vi "Assymetric_Arbitrary_Wave.vi"(9 "Time Ratios":dbl[](array[numeric]), 10 "Ub":dbl=1.0, 11 "samples":i32=128) -> (1 "offset":dbl, 2 "amplitude":dbl, 3 "Arbitary Assymetric Waveform":dbl[](array[numeric]))   [LabVIEW 2011]
uses:
  <vilib>/Analysis/baseanly.llb/Scale 1D.vi
  <vilib>/Analysis/NI_AALBase.lvlib
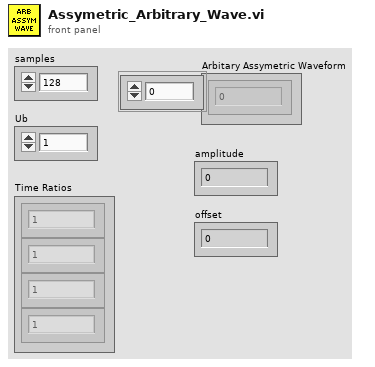
[diagram p1: front panel]
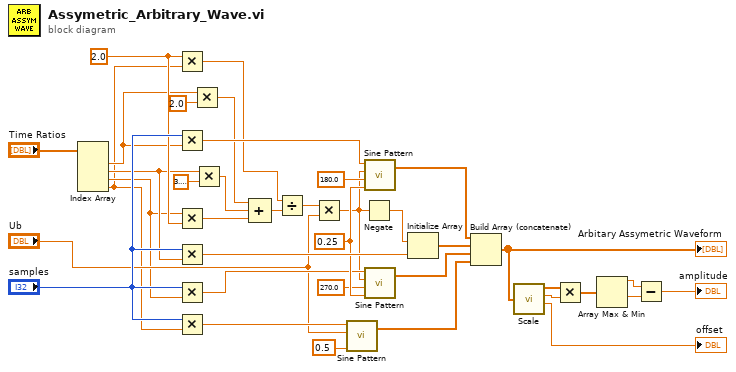
[diagram p0: block diagram]
diagram:
  w15 = 2.0 ("y")
  w33 = 0.25 ("cycles")
  n1 = Index Array(array="Time Ratios") -> (element #1=w12:dbl, element #2=w11:dbl, element #3=w10:dbl, element #4=w9:dbl)  [unwired: 4 in]
  n2 = Multiply(x=w15, y=w9) -> (x*y=w14:dbl)
  n3 = Multiply(x="samples", y=w12) -> (x*y=w36:dbl)
  n4 = Multiply(x=w10, y=w15) -> (x*y=w17:dbl)
  n5 = Multiply(x="samples", y=w11) -> (x*y=w34:dbl)
  n6 = Multiply(x="samples", y=w10) -> (x*y=w30:dbl)
  n7 = Multiply(x="samples", y=w9) -> (x*y=w38:dbl)
  n8 = Multiply(x=w12, y=2.0) -> (x*y=w22:dbl)
  n9 = Multiply(x=w11, y=3.141592653589793) -> (x*y=w21:dbl)
  n10 = Compound Arithmetic op=ADD(w22, w21, w17) -> (w20:dbl)
  n11 = Divide(x=w14, y=w20) -> (x/y=w19:dbl)
  n12 = Multiply(x=w19, y="Ub") -> (x*y=w24:dbl)
  n13 = call <vilib>:"Sine Pattern.vi"("cycles"=0.5, "amplitude"="Ub", "samples"=w38) -> ("Sinusoidal Pattern"=w26:dbl[])  [unwired: 1 in, 1 out]
  n14 = Negate(x=w24) -> (-x=w25:dbl)
  n15 = call <vilib>:"Sine Pattern.vi"("cycles"=w33, "phase(degrees)"=180.0 ("cycles"), "amplitude"=w24, "samples"=w36) -> ("Sinusoidal Pattern"=w29:dbl[])  [unwired: 1 out]
  n16 = call <vilib>:"Sine Pattern.vi"("cycles"=w33, "phase(degrees)"=270.0 ("cycles"), "amplitude"=w24, "samples"=w30) -> ("Sinusoidal Pattern"=w27:dbl[])  [unwired: 1 out]
  n17 = Initialize Array(w25, w34) -> (w28:dbl[])
  n18 = Build Array (concatenate)(w29, w28, w27, w26) -> (w1:dbl[])
  "Arbitary Assymetric Waveform" <- w1
  n19 = call-poly <vilib>:"Scale.vi"("X"=w1) -> ("Y=(X-offset)/scale"=w7:dbl[], "scale"=w8:dbl, "offset"=→"offset":dbl)  [unwired: 1 out]
  n20 = Multiply(x=w7, y=w8) -> (x*y=w6:dbl[])
  n21 = Array Max & Min(array=w6) -> (max value=w5:dbl, min value=w4:dbl)  [unwired: 2 out]
  n22 = Subtract(x=w5, y=w4) -> (x-y=→"amplitude":dbl)
